vi "Get Calibration Date.vi"(8 "error in (no error)":errorcluster, 10 "Calibration Type (0: B5725)":u32(ring) items=["B5725", "CAL", "WBFLAT", "WBGAIN", "ZERO"], 11 "VISA resource name":refnum<visa-resource-name>) -> (0 "error out":errorcluster, 1 "Month":i32, 2 "Day":i32, 3 "VISA resource name out":refnum<visa-resource-name>, 4 "Year":i32)   [LabVIEW 2014, in "Fluke 5XXX Series Multicalibrators.lvlib"]
doc: "This VI returns the date of the most recent calibration of the specified type.\n\nNote:\n\nThis VI is available only for instrument models 5700A, 5720A and 57LFC."
uses:
  Fluke 5XXX Series Multicalibrators.lvlib
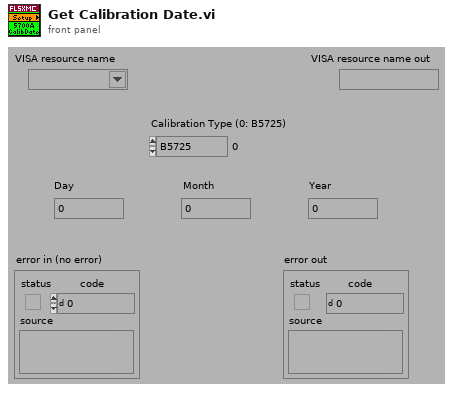
[diagram p1: front panel]
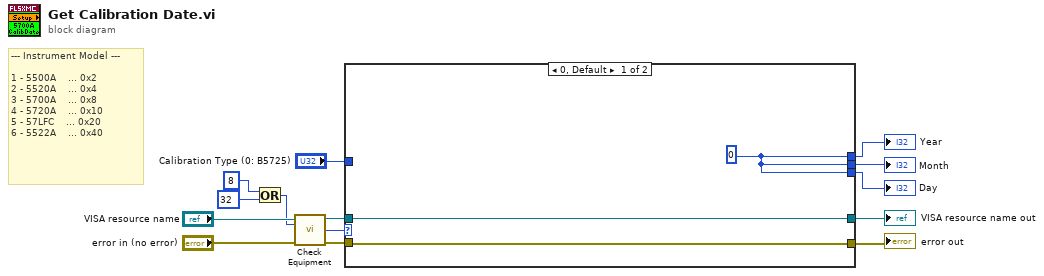
[diagram p0: block diagram]
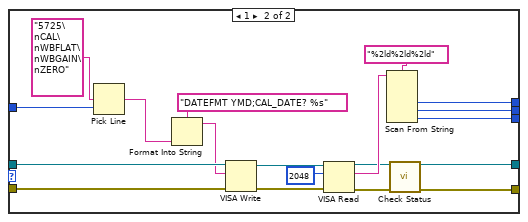
[diagram p2: hidden frame]
diagram:
  # "--- Instrument Model ---\n\n1 - 5500A    ... 0x2\n2 - 5520A    ... 0x4\n3 - 5700A    ... 0x8\n4 - 5720A    ... 0x10\n5 - 57LFC    ... 0x20\n6 - 5522A    ... 0x40"
  n1 = Or(x=8 ("Numeric"), y=32 ("Numeric")) -> (x .or. y?=w7:i32)
  n2 = call "Check Equipment.vi"("error in (no error)"="error in (no error)", "Bit Mask"=w7, "VISA resource name"="VISA resource name") -> ("error out"=w10:errorcluster, "Present?"=w8:u32, "VISA resource name out"=w9:refnum<visa-resource-name>)  [unwired: 6 in]
  n3 = case shown="0, Default" w8 {
    tunnel: w10 -> [w16 w35]
    tunnel: w9 -> [w17 w34]
    tunnel: "Calibration Type (0: B5725)" -> [_ w33]
    tunnel: [w16 w23] -> w5
    tunnel: [w17 w22] -> w4
    tunnel: [w15 w21] -> w3
    tunnel: [w15 w20] -> w2
    tunnel: [w15 w19] -> w1
    frame 0, Default {
      w15 = 0
    }
    frame 1 {
      n4 = Pick Line(multi-line string="5725\nCAL\nWBFLAT\nWBGAIN\nZERO", line index=w33) -> (output string=w18:string)  [unwired: 1 in]
      n5 = Format Into String(format string="DATEFMT YMD;CAL_DATE? %s" ("Reset Command"), w18) -> (resulting string=w31:string)  [unwired: 2 in, 1 out]
      n6 = VISA Write(VISA resource name=w34, write buffer=w31, error in (no error)=w35) -> (VISA resource name out=w27:refnum<visa-resource-name>, error out=w26:errorcluster)  [unwired: 1 out]
      n7 = VISA Read(VISA resource name=w27, byte count=u32 2048 ("byte count (0)"), error in (no error)=w26) -> (VISA resource name out=w24:refnum<visa-resource-name>, read buffer=w28:string, error out=w25:errorcluster)  [unwired: 1 out]
      n8 = Scan From String(format string="%2ld%2ld%2ld", input string=w28) -> (output 1=w21:i32, output 2=w20:i32, output 3=w19:i32)  [unwired: 5 in, 3 out]
      n9 = call "Check Status.vi"("VISA resource name"=w24, "error in (no error)"=w25) -> ("VISA resource name out"=w22:refnum<visa-resource-name>, "error out"=w23:errorcluster)  [unwired: 12 in]
    }
  }
  "Day" <- w1
  "Month" <- w2
  "Year" <- w3
  "VISA resource name out" <- w4
  "error out" <- w5
